vi "MessungHystereseschleife.vi"(7 "Messung Hystereseschleife":T3, 8 "Error in":errorcluster, 9 "Globale Variablen":T1, 10 "GUI Data":T4={"Eisenquerschnitt [mm^2]"=45.0, "Wirksame Länge [cm]"=94.0, "Primärwindungszahl"=700.0, "Sekundärwindungszahl"=700.0, "Messwiderstand [Ohm]"=1.0, "Spannungsteilerverhaeltnis (1/x)"=1.0, "Probenbezeichnung"="", "Dichte des Eisens [g/cm^3]"=7.0, "magn. Flussdichte [T]"=2.0, "Frequenz [Hz]"=50.0, "Namen"="", "Gruppe"=""}, 11 "GUI Einstellungen":T2) -> (0 "Error out":errorcluster, 1 "Globale Variablen out":T1, 2 "GUI Data out":T4, 3 "GUI Einstellungen out":T2, 5 "Messung Hystereseschleife out":T3)   [LabVIEW 2016]
doc: "Nimmt die nach der Flussdichte-Anpassungs.vi detektierten Einstellungen um die Hystereseschleife zu messen. Es wird ebenfalls die Remanenz und Koerzitivfeldstaerke bestimmt."
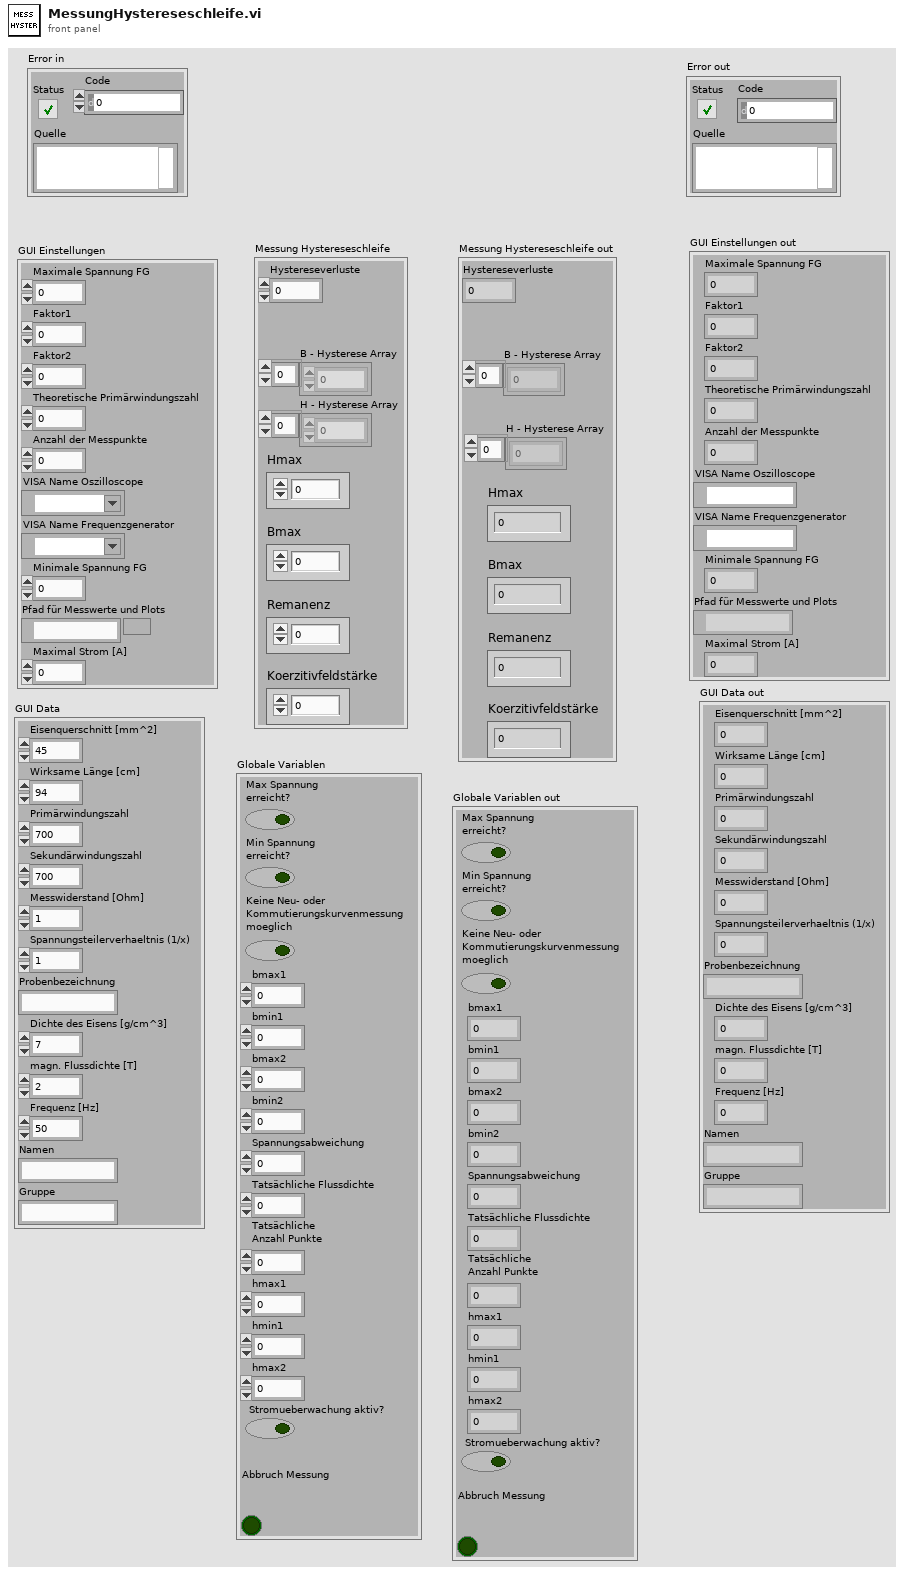
[diagram p1: front panel]
types:
  T1 = cluster{"Max Spannung\nerreicht?":bool, "Min Spannung\nerreicht?":bool, "Keine Neu- oder\nKommutierungskurvenmessung\nmoeglich":bool, "bmax1":dbl, "bmin1":dbl, "bmax2":dbl, "bmin2":dbl, "Spannungsabweichung":dbl, "Tatsächliche Flussdichte":dbl, "Tatsächliche \nAnzahl Punkte":dbl, "hmax1":dbl, "hmin1":dbl, "hmax2":dbl, " Stromueberwachung aktiv?":bool, "Abbruch Messung":bool}
  T2 = cluster{"Maximale Spannung FG":dbl, "Faktor1":dbl, "Faktor2":dbl, "Theoretische Primärwindungszahl":dbl, "Anzahl der Messpunkte":i32, "VISA Name Oszilloscope":refnum<visa-resource-name>, "VISA Name Frequenzgenerator":refnum<visa-resource-name>, "Minimale Spannung FG":dbl, "Pfad für Messwerte und Plots":path, "Maximal Strom [A] ":dbl}
  T3 = cluster{"Hystereseverluste":dbl, "B - Hysterese Array":dbl[], "H - Hysterese Array":dbl[], "Hmax":dbl, "Bmax":dbl, "Remanenz":dbl, "Koerzitivfeldstärke":dbl}
  T4 = cluster{"Eisenquerschnitt [mm^2]":dbl, "Wirksame Länge [cm]":dbl, "Primärwindungszahl":dbl, "Sekundärwindungszahl":dbl, "Messwiderstand [Ohm]":dbl, "Spannungsteilerverhaeltnis (1/x)":dbl, "Probenbezeichnung":string, "Dichte des Eisens [g/cm^3]":dbl, "magn. Flussdichte [T]":dbl, "Frequenz [Hz]":dbl, "Namen":string, "Gruppe":string}
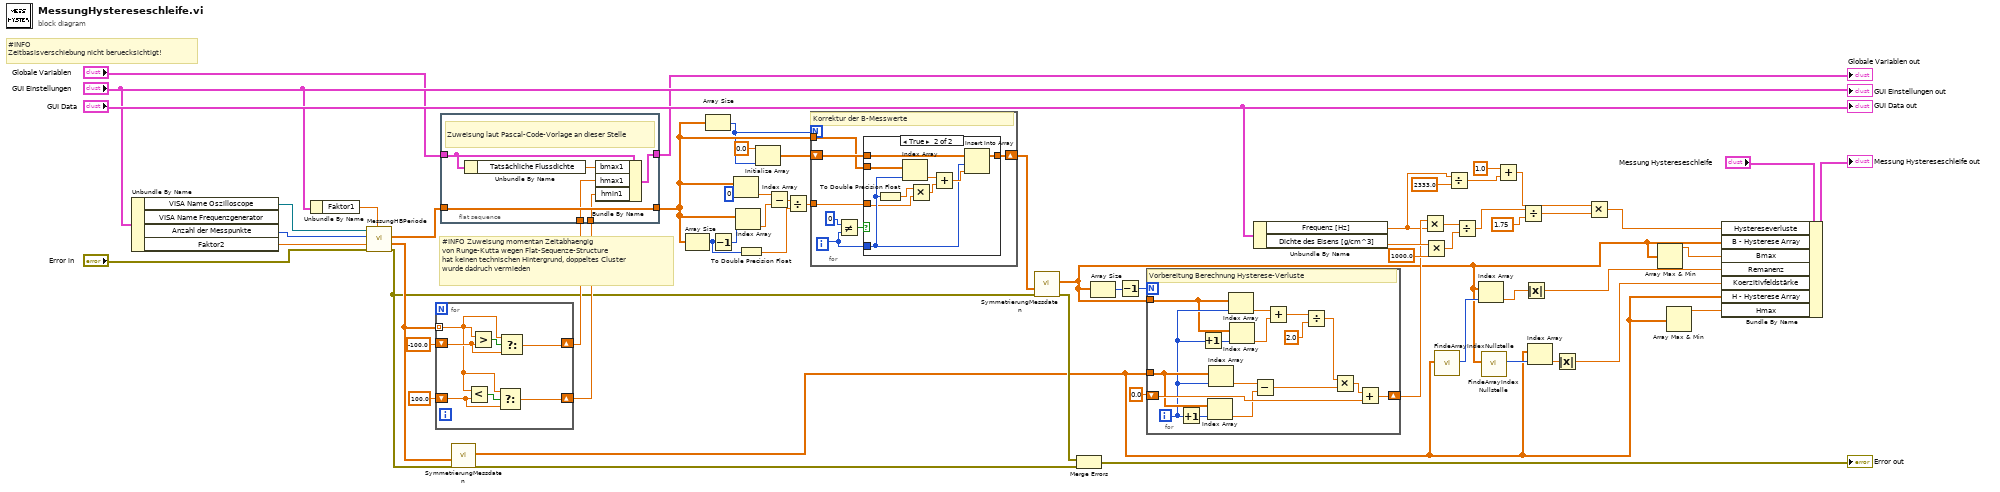
[diagram p0: block diagram]
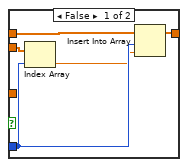
[diagram p2: hidden frame]
diagram:
  # "#INFO\nZeitbasisverschiebung nicht beruecksichtigt!"
  # "#INFO Zuweisung momentan Zeitabhaengig\nvon Runge-Kutta wegen Flat-Sequenze-Structure\nhat keinen technischen Hintergrund, doppeltes Cluster\nwurde dadruch vermieden"
  n1 = Unbundle By Name("GUI Einstellungen") -> ("VISA Name Oszilloscope"=w37:refnum<visa-resource-name>, "Anzahl der Messpunkte"=w36:i32, "Faktor2"=w35:dbl)  [unwired: 1 out]
  n2 = Unbundle By Name("GUI Einstellungen") -> ("Faktor1"=w33:dbl)
  n3 = call "MessungHBPeriode.vi"("Faktor 1"=w33, "Error_in"="Error in", "Faktor2 (1)"=w35, "Anzahl der Messpunkte"=w36, "VISA Name OZ in(OZ)"=w37) -> ("Error_out"=w31:errorcluster, "H-Messdaten einer periode"=w34:dbl[], "B-Messdaten einer periode"=w32:dbl[])  [unwired: 3 in, 1 out]
  n4 = for {
    shift-right: [w67] -> w40
    shift-left: -100.0 -> [w68]
    shift-right: [w64] -> w39
    shift-left: 100.0 -> [w63]
    tunnel: w34 -> [w62] mode=indexing
    n5 = Less?(x=w62, y=w63) -> (x < y?=w65:bool)
    n6 = Greater?(x=w62, y=w68) -> (0:w66:bool)
    n7 = Select(t=w62, s=w65, f=w63) -> (s? t:f=w64:dbl)
    n8 = Select(t=w62, s=w66, f=w68) -> (s? t:f=w67:dbl)
  }
  n9 = flat-sequence {
    tunnel: w32 -> [w74]
    tunnel: [w74] -> w30
    tunnel: "Globale Variablen" -> [w72]
    tunnel: [w73] -> w12
    tunnel: w40 -> [w70]
    tunnel: w39 -> [w69]
    frame #0 {
      # "Zuweisung laut Pascal-Code-Vorlage an dieser Stelle"
      n10 = Unbundle By Name(w72) -> ("Tatsächliche Flussdichte"=w71:dbl)
      n11 = Bundle By Name(cluster=w72, "bmax1"=w71, "hmax1"=w70, "hmin1"=w69) -> (w73:T1)
    }
  }
  n12 = call "SymmetrierungMessdaten.vi"("error in"=w31, "Input Array"=w34) -> ("error out"=w46:errorcluster, "Output Array"=w11:dbl[])  [unwired: 3 in, 3 out]
  n13 = Array Size(array=w30) -> (size(s)=w54:i32)
  n14 = Array Size(array=w30) -> (size(s)=w26:i32)
  n15 = Decrement(x=w54) -> (x-1=w56:i32)
  n16 = Index Array(array=w30, index=0) -> (element=w58:dbl)
  n17 = Index Array(array=w30, index=w56) -> (element=w57:dbl)
  n18 = To Double Precision Float(number=w54) -> (double precision float=w53:dbl)
  n19 = Initialize Array(0.0 ("element"), w26) -> (w28:dbl[])
  n20 = Subtract(x=w58, y=w57) -> (x-y=w55:dbl)
  n21 = Divide(x=w55, y=w53) -> (x/y=w19:dbl)
  n22 = for {
    N: w26 -> [_]
    tunnel: w30 -> [w76]
    shift-right: [w77] -> w29
    shift-left: w28 -> [w78]
    tunnel: w19 -> [w75]
    i -> [w79]
    # "Korrektur der B-Messwerte"
    n23 = Not Equal?(x=0, y=w79) -> (x != y?=w80:bool)
    n24 = case shown="True" w80 {
      tunnel: w78 -> [w85 w95]
      tunnel: w79 -> [w83 w88]
      tunnel: [w86 w94] -> w77
      tunnel: w76 -> [w84 w93]
      tunnel: w75 -> [_ w87]
      frame False {
        n25 = Index Array(array=w84, index=w83) -> (element=w82:dbl)
        n26 = Insert Into Array(array=w85, index=w83, new element=w82) -> (w86:dbl[])
      }
      frame True {
        n27 = To Double Precision Float(number=w88) -> (double precision float=w90:dbl)
        n28 = Index Array(array=w93, index=w88) -> (element=w92:dbl)
        n29 = Multiply(x=w90, y=w87) -> (x*y=w91:dbl)
        n30 = Add(x=w92, y=w91) -> (x+y=w89:dbl)
        n31 = Insert Into Array(array=w95, index=w88, new element=w89) -> (w94:dbl[])
      }
    }
  }
  n32 = call "SymmetrierungMessdaten.vi"("error in"=w31, "Input Array"=w29) -> ("error out"=w18:errorcluster, "Output Array"=w10:dbl[])  [unwired: 3 in, 3 out]
  n33 = Merge Errors(w18, w46) -> (→"Error out":errorcluster)
  n34 = Array Size(array=w10) -> (size(s)=w52:i32)
  n35 = Decrement(x=w52) -> (x-1=w51:i32)
  n36 = for {
    N: w51 -> [_]
    tunnel: w10 -> [w101]
    shift-right: [w110] -> w17
    shift-left: 0.0 -> [w111]
    tunnel: w11 -> [w108]
    i -> [w102]
    # "Vorbereitung Berechnung Hysterese-Verluste"
    n37 = Increment(x=w102) -> (x+1=w107:i32)
    n38 = Increment(x=w102) -> (x+1=w103:i32)
    n39 = Index Array(array=w108, index=w107) -> (element=w106:dbl)
    n40 = Index Array(array=w108, index=w102) -> (element=w109:dbl)
    n41 = Index Array(array=w101, index=w102) -> (element=w104:dbl)
    n42 = Index Array(array=w101, index=w103) -> (element=w100:dbl)
    n43 = Subtract(x=w109, y=w106) -> (x-y=w105:dbl)
    n44 = Add(x=w104, y=w100) -> (x+y=w99:dbl)
    n45 = Divide(x=w99, y=2.0 ("Schwaderersche\nKonstante")) -> (x/y=w97:dbl)
    n46 = Multiply(x=w97, y=w105) -> (x*y=w96:dbl)
    n47 = Add(x=w96, y=w111) -> (x+y=w110:dbl)
  }
  n48 = Unbundle By Name("GUI Data") -> ("Frequenz [Hz]"=w1:dbl, "Dichte des Eisens [g/cm^3]"=w43:dbl)
  n49 = Multiply(x=w17, y=w1) -> (x*y=w49:dbl)
  n50 = Multiply(x=w43, y=1000.0) -> (x*y=w47:dbl)
  n51 = call "FindeArrayIndexNullstelle.vi"("Array"=w11) -> ("Array Index Nullstelle"=w16:i32)  [unwired: 10 in]
  n52 = Divide(x=w1, y=2333.0) -> (x/y=w3:dbl)
  n53 = Divide(x=w49, y=w47) -> (x/y=w8:dbl)
  n54 = Index Array(array=w10, index=w16) -> (element=w22:dbl)
  n55 = call "FindeArrayIndexNullstelle.vi"("Array"=w10) -> ("Array Index Nullstelle"=w15:i32)  [unwired: 10 in]
  n56 = Add(x=1.0, y=w3) -> (x+y=w4:dbl)
  n57 = Divide(x=w8, y=1.75 ("Schwaderersche\nKonstante")) -> (x/y=w7:dbl)
  n58 = Absolute Value(x=w22) -> (abs(x)=w14:dbl)
  n59 = Index Array(array=w11, index=w15) -> (element=w21:dbl)
  n60 = Absolute Value(x=w21) -> (abs(x)=w20:dbl)
  n61 = Multiply(x=w4, y=w7) -> (x*y=w6:dbl)
  n62 = Array Max & Min(array=w10) -> (max value=w23:dbl)  [unwired: 3 out]
  n63 = Array Max & Min(array=w11) -> (max value=w24:dbl)  [unwired: 3 out]
  n64 = Bundle By Name(cluster="Messung Hystereseschleife", "Hystereseverluste"=w6, "B - Hysterese Array"=w10, "Bmax"=w23, "Remanenz"=w14, "Koerzitivfeldstärke"=w20, "H - Hysterese Array"=w11, "Hmax"=w24) -> (→"Messung Hystereseschleife out":T3)
  "GUI Data out" <- "GUI Data"
  "GUI Einstellungen out" <- "GUI Einstellungen"
  "Globale Variablen out" <- w12
